vi "第3題.vi"() -> ()   [LabVIEW 2017]
uses:
  <vilib>/Utility/file.llb/Read Delimited Spreadsheet (DBL).vi
panel:
  in  "取幾小時數據":i32
  in  "幾點開始":i32
  out "S是否有偏群":bool
  out "Q是否有偏群":bool
  out "S可能群數":dbl
  out "Q可能偏群數":dbl
  out "size(s)":i32
  in  "file path (dialog if empty)":path
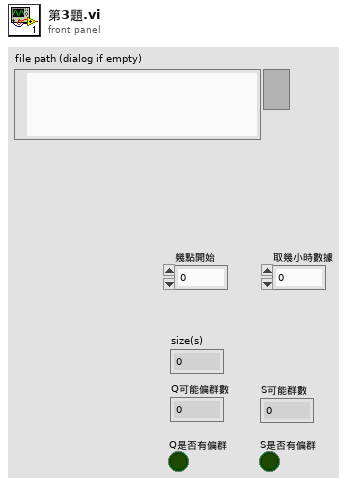
[diagram p1: front panel]
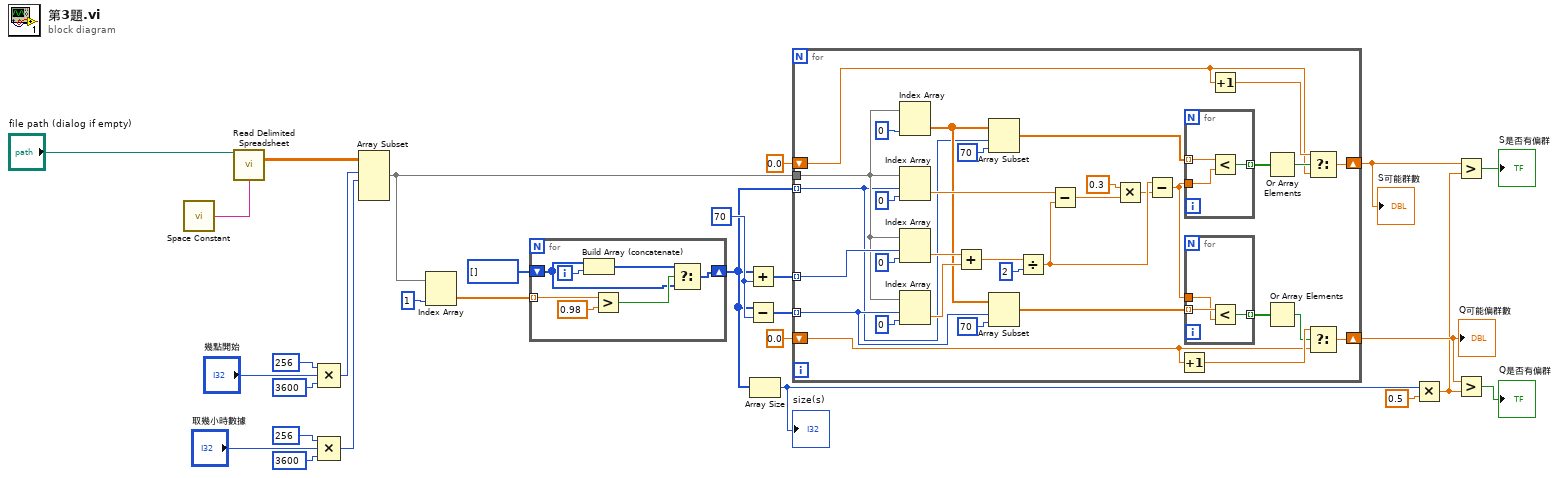
[diagram p0: block diagram]
diagram:
  w22 = 70
  n1 = call <vilib>:"Space Constant.vi"() -> ("String"=w27:string)
  n2 = call-poly <vilib>:"Read Delimited Spreadsheet.vi"("file path (dialog if empty)"="file path (dialog if empty)", "delimiter (\\t)"=w27) -> ("all rows"=w26:dbl[][])  [unwired: 8 in, 5 out]
  n3 = Compound Arithmetic op=MULTIPLY(256, "幾點開始", 3600) -> (w8:i32)
  n4 = Compound Arithmetic op=MULTIPLY(256, "取幾小時數據", 3600) -> (w4:i32)
  n5 = Array Subset(array=w26, index (row)=w8, length (row)=w4) -> (w19:dbl[][])  [unwired: 2 in]
  n6 = Index Array(array=w19, index (col)=1 ("disabled index (col)")) -> (element=w24:dbl[])  [unwired: 1 in]
  n7 = for {
    tunnel: w24 -> [w34] mode=indexing
    shift-right: [w32] -> w18
    shift-left: i32[] [] -> [w29]
    i -> [w30]
    n8 = Build Array (concatenate)(w29, w30) -> (w31:i32[])
    n9 = Greater?(x=w34, y=0.98) -> (0:w33:bool)
    n10 = Select(t=w31, s=w33, f=w29) -> (s? t:f=w32:i32[])
  }
  n11 = Add(x=w18, y=w22) -> (x+y=w21:i32[])
  n12 = Subtract(x=w18, y=w22) -> (x-y=w20:i32[])
  n13 = Array Size(array=w18) -> (size(s)=w17:i32)
  "size(s)" <- w17
  n14 = for {
    tunnel: w21 -> [w66] mode=indexing
    tunnel: w20 -> [w53] mode=indexing
    tunnel: w19 -> [w58]
    tunnel: w18 -> [w40] mode=indexing
    shift-right: [w47] -> w13
    shift-left: 0.0 -> [w46]
    shift-right: [w36] -> w12
    shift-left: 0.0 -> [w37]
    n15 = Index Array(array=w58, index (col)=0 ("disabled index (col)")) -> (element=w41:dbl[])  [unwired: 1 in]
    n16 = Index Array(array=w58, index (row)=w40, index (col)=0 ("disabled index (col)")) -> (element=w56:dbl)
    n17 = Index Array(array=w58, index (row)=w66, index (col)=0 ("disabled index (col)")) -> (element=w65:dbl)
    n18 = Index Array(array=w58, index (row)=w53, index (col)=0 ("disabled index (col)")) -> (element=w64:dbl)
    n19 = Add(x=w65, y=w64) -> (x+y=w63:dbl)
    n20 = Array Subset(array=w41, index=w40, length=70) -> (w39:dbl[])
    n21 = Array Subset(array=w41, index=w53, length=70) -> (w51:dbl[])
    n22 = Divide(x=w63, y=2) -> (x/y=w55:dbl)
    n23 = Subtract(x=w56, y=w55) -> (x-y=w60:dbl)
    n24 = Multiply(x=0.3, y=w60) -> (x*y=w54:dbl)
    n25 = Subtract(x=w55, y=w54) -> (x-y=w38:dbl)
    n26 = Increment(x=w46) -> (x+1=w49:dbl)
    n27 = for {
      tunnel: w38 -> [w70]
      tunnel: w39 -> [w71] mode=indexing
      tunnel: [w69] -> w45 mode=indexing
      n28 = Less?(x=w71, y=w70) -> (x < y?=w69:bool)
    }
    n29 = for {
      tunnel: w38 -> [w73]
      tunnel: w51 -> [w74] mode=indexing
      tunnel: [w72] -> w50 mode=indexing
      n30 = Less?(x=w74, y=w73) -> (x < y?=w72:bool)
    }
    n31 = Increment(x=w37) -> (x+1=w44:dbl)
    n32 = Or Array Elements(Boolean array=w45) -> (logical OR=w43:bool)
    n33 = Or Array Elements(Boolean array=w50) -> (logical OR=w48:bool)
    n34 = Select(t=w44, s=w43, f=w37) -> (s? t:f=w36:dbl)
    n35 = Select(t=w49, s=w48, f=w46) -> (s? t:f=w47:dbl)
  }
  "Q可能偏群數" <- w13
  "S可能群數" <- w12
  n36 = Multiply(x=w17, y=0.5) -> (x*y=w3:dbl)
  n37 = Greater?(x=w12, y=w3) -> (0:→"S是否有偏群":bool)
  n38 = Greater?(x=w13, y=w3) -> (0:→"Q是否有偏群":bool)
